vi "Init Image Display (SubVI).vi"(8 "error in":errorcluster, 11 "Variant":variant) -> (0 "error out":errorcluster)   [LabVIEW 2012]
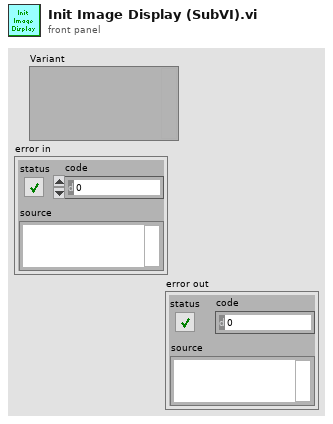
[diagram p1: front panel]
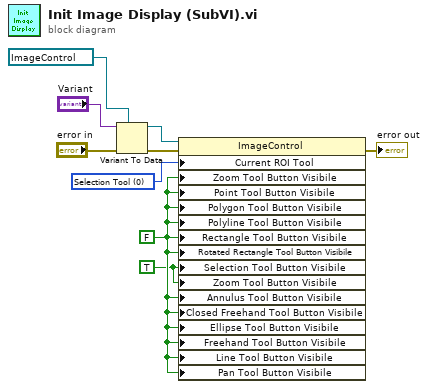
[diagram p0: block diagram]
diagram:
  w5 = TRUE ("ROI Tool Buttons Visibile:Zoom Tool Button Visible")
  w6 = FALSE ("ROI Tool Buttons Visibile:Zoom Tool Button Visible")
  w4 = u32 0 items=["Zoom Tool"=8, "Selection Tool"=0, "Pan Tool"=9, "Point Tool"=1, "Line Tool"=2, "Rectangle Tool"=3, "Rotated Rectangle Tool"=12, "Polyline Tool"=10, "Polygon Tool"=5, "Freehand Tool"=11, "Closed Freehand Tool"=6, "Ellipse Tool"=4, "Annulus Tool"=7] ("Current ROI Tool")
  n1 = Variant To Data(error in="error in", type=refnum<vi> refnum ("Monitor image"), Variant="Variant") -> (data=w9:refnum<vi>, error out=w2:errorcluster)
  n2 = property on="Property Node" class="ImageControl"(reference=w9, error in=w2, "Current ROI Tool"=w4, "Zoom Tool Button Visibile"=w6, "Point Tool Button Visibile"=w6, "Polygon Tool Button Visibile"=w6, "Polyline Tool Button Visibile"=w6, "Rectangle Tool Button Visibile"=w6, "Rotated Rectangle Tool Button Visibile"=w6, "Selection Tool Button Visibile"=w5, "Zoom Tool Button Visibile"=w5, "Annulus Tool Button Visibile"=w6, "Closed Freehand Tool Button Visibile"=w6, "Ellipse Tool Button Visibile"=w6, "Freehand Tool Button Visibile"=w6, "Line Tool Button Visibile"=w6, "Pan Tool Button Visibile"=w6) -> (error out=→"error out":errorcluster)  [unwired: 1 out]
